vi "data check intensity_dataset-all-in-one-file.vi"() -> ()   [LabVIEW 2016]
uses:
  <vilib>/Utility/file.llb/Read Delimited Spreadsheet (DBL).vi
panel:
  in  "비활성화된 인덱스 (열)":i32
  out "크기":i32[](array[numeric])
  in  "file path (dialog if empty)":path caption="파일 경로(비었을 경우 대화 상자 창)"
  out "강도 그래프":dbl[][](graph)
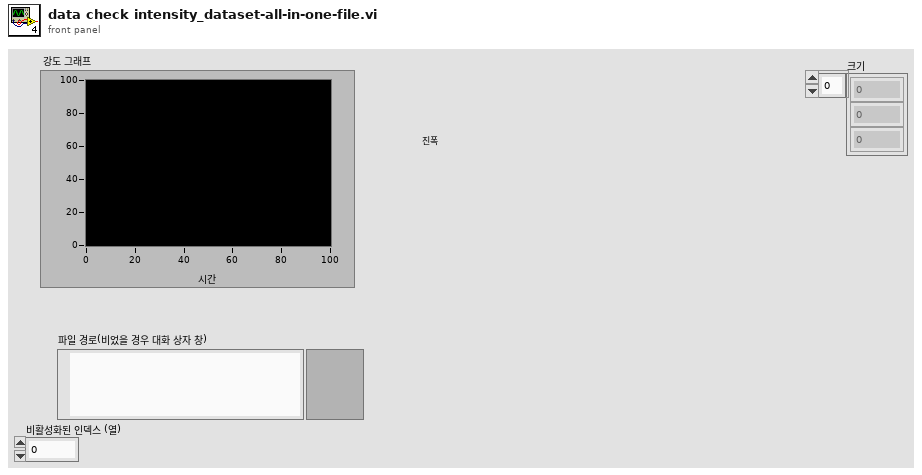
[diagram p1: front panel]
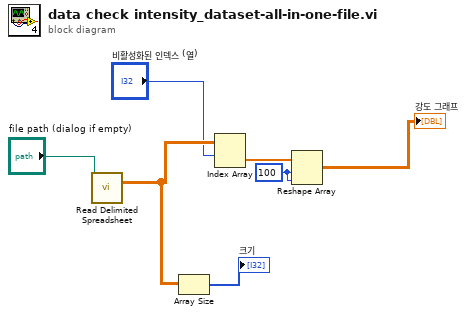
[diagram p0: block diagram]
diagram:
  w3 = 100 ("차원 크기")
  n1 = call-poly <vilib>:"Read Delimited Spreadsheet.vi"("file path (dialog if empty)"="file path (dialog if empty)") -> ("all rows"=w5:dbl[][])  [unwired: 9 in, 5 out]
  n2 = Array Size(array=w5) -> (size(s)=→"크기":i32[])
  n3 = Index Array(array=w5, index (row)="비활성화된 인덱스 (열)") -> (element=w4:dbl[])  [unwired: 1 in]
  n4 = Reshape Array(w4, w3, w3) -> (→"강도 그래프":dbl[][])
